vi "Actor Core.vi"(8 "error in":errorcluster, 11 "State in":refnum<class "Command Processor.lvclass">) -> (0 "error out":errorcluster, 3 "Actor out":refnum<class "Actor.lvclass">)   [LabVIEW 2013, in "Command Processor.lvlib" / "Command Processor.lvclass"]
doc: "(<B>Filename</B>: Actor Framework.lvlib:Actor.lvclass:Actor Core.vi)\n\nThis override invokes Entry.vi on the initial state, prior to calling the parent Actor Core. Adding this behavior to Actor Core (instead of an override of Pre Launch Init.vi) allows the initial state to launch a nested actor as part of its entry behavior.\n\nReceives messages to the actor, reacts to them, and initiates any error handling that may shut the actor down.\n\nDescendant classes may override this VI to append parallel tasks for the actor to complete while it handles messages. Overrides use the Call Parent Method node."
uses:
  Command Processor.lvclass
  <vilib>/ni/Actors/State Actor/State Actor/State Actor.lvclass
  <vilib>/ActorFramework/Actor/Actor.lvclass
  Command/Command Status.ctl
  Command/Command.lvclass
  Command/State Status.ctl
  Command Processor Status.ctl
  State Status.ctl
  Current Previous State Status.ctl
panel:
  in  "Command Processor Status":T1
  in  "Command Status":T4
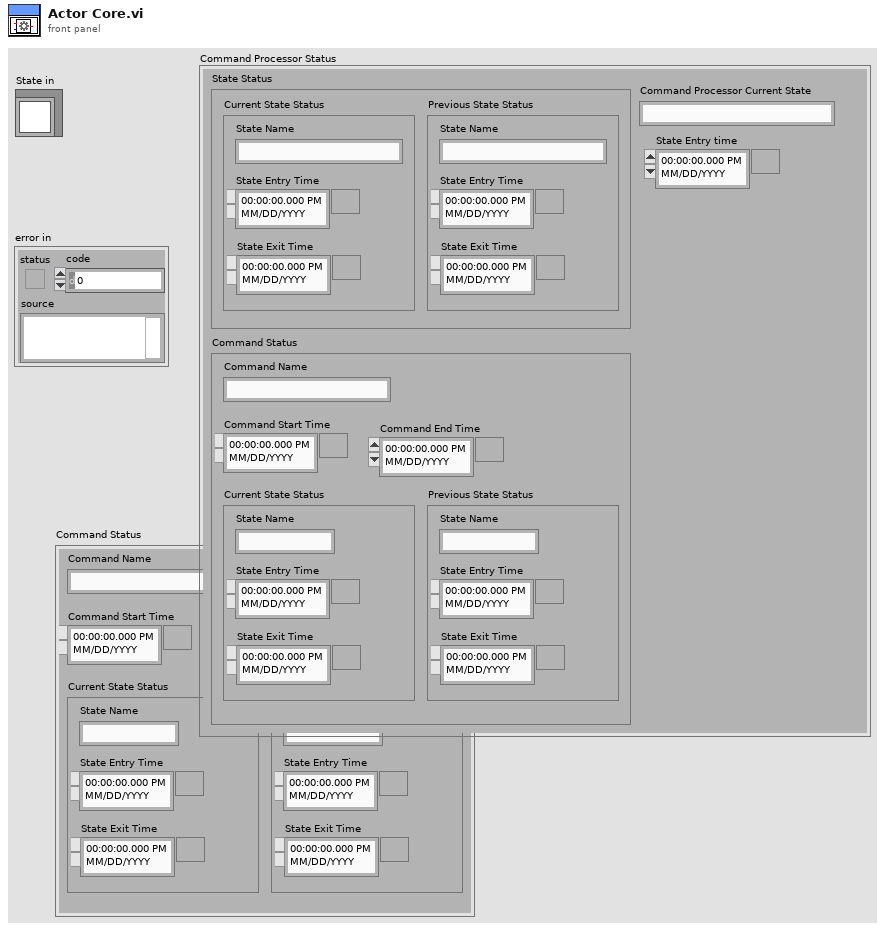
[diagram p1: front panel]
types:
  T1 = typedef "Command Processor.lvlib/Command Processor.lvclass/Command Processor Status.ctl" = cluster{"State Entry time":timestamp, "State Status":T2, "Command Processor Current State":string, "Command Status":T4}
  T2 = typedef "Current Previous State Status.ctl" = cluster{"Current State Status":T3, "Previous State Status":T3}
  T3 = typedef "State Status.ctl" = cluster{"State Name":string, "State Entry Time":timestamp, "State Exit Time":timestamp}
  T4 = typedef "Command Processor.lvlib/Command.lvlib/Command.lvclass/Command Status.ctl" = cluster{"Command Name":string, "Current State Status":T5, "Command Start Time":timestamp, "Command End Time":timestamp, "Previous State Status":T5}
  T5 = typedef "Command Processor.lvlib/Command.lvlib/Command.lvclass/State Status.ctl" = cluster{"State Name":string, "State Entry Time":timestamp, "State Exit Time":timestamp}
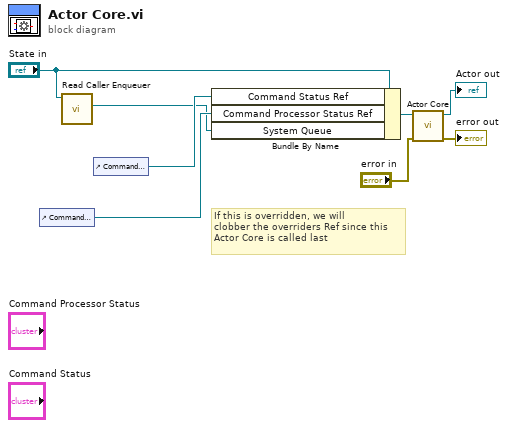
[diagram p0: block diagram]
diagram:
  # "If this is overridden, we will\nclobber the overriders Ref since this \nActor Core is called last"
  n1 = control-ref of="Command Processor Status"() -> (w3:refnum<vi>)
  n2 = call <vilib>:"Read Caller Enqueuer.vi"("Actor"="State in") -> ("Caller Enqueuer"=w1:refnum<class "Message Enqueuer.lvclass">)  [unwired: 10 in]
  n3 = control-ref of="Command Status"() -> (w4:refnum<vi>)
  n4 = Bundle By Name(cluster="State in", "Command Status Ref"=w4, "Command Processor Status Ref"=w3, "System Queue"=w1) -> (w5:refnum<class "Command Processor.lvclass">)
  n5 = call-parent "Actor Core.vi"("error in"="error in", "State in"=w5) -> ("error out"=→"error out":errorcluster, "Actor out"=→"Actor out":refnum<class "Actor.lvclass">)  [unwired: 8 in]
